vi "_AllThings.vi"   [LabVIEW 2024]
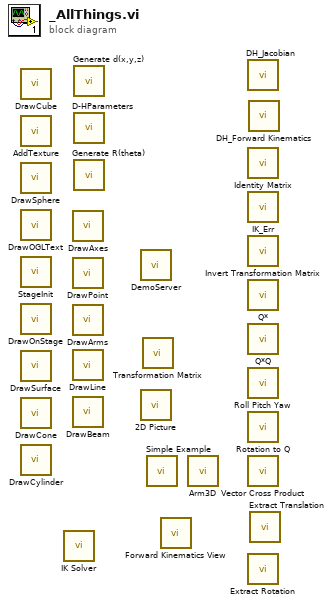
[diagram p0: block diagram]
diagram:
  n1 = call <userlib>:"DrawCube.vi"() -> ()  [unwired: 6 in, 2 out]
  n2 = call <userlib>:"AddTexture.vi"() -> ()  [unwired: 4 in, 2 out]
  n3 = call <userlib>:"DrawSphere.vi"() -> ()  [unwired: 6 in, 2 out]
  n4 = call <userlib>:"DrawOGLText.vi"() -> ()  [unwired: 6 in, 2 out]
  n5 = call <userlib>:"StageInit.vi"() -> ()  [unwired: 4 in, 2 out]
  n6 = call <userlib>:"DrawOnStage.vi"() -> ()  [unwired: 3 in, 3 out]
  n7 = call <userlib>:"DrawSurface.vi"() -> ()  [unwired: 6 in, 2 out]
  n8 = call <userlib>:"DrawCone.vi"() -> ()  [unwired: 6 in, 2 out]
  n9 = call <userlib>:"DrawCylinder.vi"() -> ()  [unwired: 6 in, 2 out]
  n10 = call <userlib>:"IK Solver.vi"() -> ()  [unwired: 12 in]
  n11 = call <userlib>:"DrawAxes.vi"() -> ()  [unwired: 5 in, 1 out]
  n12 = call <userlib>:"DrawPoint.vi"() -> ()  [unwired: 3 in, 1 out]
  n13 = call <userlib>:"DrawArms.vi"() -> ()  [unwired: 6 in, 2 out]
  n14 = call <userlib>:"DrawLine.vi"() -> ()  [unwired: 5 in, 2 out]
  n15 = call <userlib>:"DrawBeam.vi"() -> ()  [unwired: 6 in, 1 out]
  n16 = call <userlib>:"Generate d(x,y,z).vi"() -> ()  [unwired: 3 in, 1 out]
  n17 = call <userlib>:"D-HParameters.vi"() -> ()  [unwired: 2 in, 2 out]
  n18 = call <userlib>:"Generate R(theta).vi"() -> ()  [unwired: 3 in, 1 out]
  n19 = call <userlib>:"DemoServer.vi"() -> ()  [unwired: 12 in]
  n20 = call <userlib>:"2D Picture.vi"() -> ()  [unwired: 11 in, 1 out]
  n21 = call <userlib>:"Transformation Matrix.vi"() -> ()  [unwired: 11 in, 1 out]
  n22 = call <userlib>:"Simple Example.vi"() -> ()  [unwired: 12 in]
  n23 = call <userlib>:"Forward Kinematics View.vi"() -> ()  [unwired: 10 in, 2 out]
  n24 = call <userlib>:"Arm3D.vi"() -> ()  [unwired: 12 in]
  n25 = call <userlib>:"DH_Jacobian.vi"() -> ()  [unwired: 2 in, 2 out]
  n26 = call <userlib>:"Identity Matrix.vi"() -> ()  [unwired: 1 in, 1 out]
  n27 = call <userlib>:"IK_Err.vi"() -> ()  [unwired: 3 in, 1 out]
  n28 = call <userlib>:"Invert Transformation Matrix.vi"() -> ()  [unwired: 1 in, 1 out]
  n29 = call <userlib>:"Q*.vi"() -> ()  [unwired: 1 in, 1 out]
  n30 = call <userlib>:"Q*Q.vi"() -> ()  [unwired: 3 in, 1 out]
  n31 = call <userlib>:"Roll Pitch Yaw.vi"() -> ()  [unwired: 1 in, 1 out]
  n32 = call <userlib>:"Rotation to Q.vi"() -> ()  [unwired: 1 in, 1 out]
  n33 = call <userlib>:"Vector Cross Product.vi"() -> ()  [unwired: 3 in, 1 out]
  n34 = call <userlib>:"Extract Rotation.vi"() -> ()  [unwired: 1 in, 1 out]
  n35 = call <userlib>:"DH_Forward Kinematics.vi"() -> ()  [unwired: 4 in, 4 out]
  n36 = call <userlib>:"Extract Translation.vi"() -> ()  [unwired: 1 in, 1 out]
